vi "StrError.vi"(8 "error in (no error)":errorcluster, 10 "errnum":i32, 11 "modbus in":refnum<class "libmodbus.lvclass">) -> (0 "error out":errorcluster, 2 "error message":string, 3 "modbus out":refnum<class "libmodbus.lvclass">)   [LabVIEW 2017, in "libmodbus.lvlib" / "libmodbus.lvclass"]
doc: "Retuns the error message for <b>errnum</b>."
uses:
  libmodbus.lvclass
  libmodbus.lvclass/libmodbus.ctl
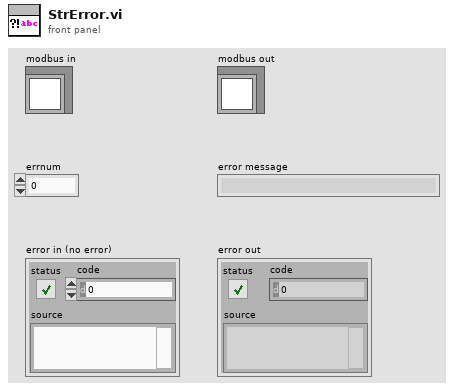
[diagram p1: front panel]
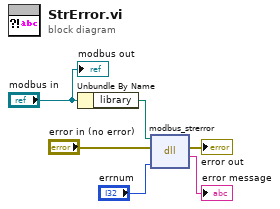
[diagram p0: block diagram]
diagram:
  n1 = Unbundle By Name("modbus in") -> ("library"=w5:path)
  n2 = dll-call lib="?" fn="modbus_strerror"(path in=w5, error in="error in (no error)", "errnum"="errnum") -> (error out=→"error out":errorcluster, "char"=→"error message":string)  [unwired: 2 in, 1 out]
  "modbus out" <- "modbus in"
